vi "instert_before.vi"(8 "error in (no error)":errorcluster, 9 "current node":refnum<class "Iterator.lvclass">, 10 "data":variant, 11 "DoublyLinkedList in":refnum<class "DoublyLinkedList.lvclass">) -> (0 "error out":errorcluster, 3 "DoublyLinkedList out":refnum<class "DoublyLinkedList.lvclass">)   [LabVIEW 2021, in "DoublyLinkedList.lvclass"]
uses:
  DoublyLinkedList.lvclass
  Iterator/Iterator.lvclass
  DoublyLinkedList.lvclass/DoublyLinkedList.ctl
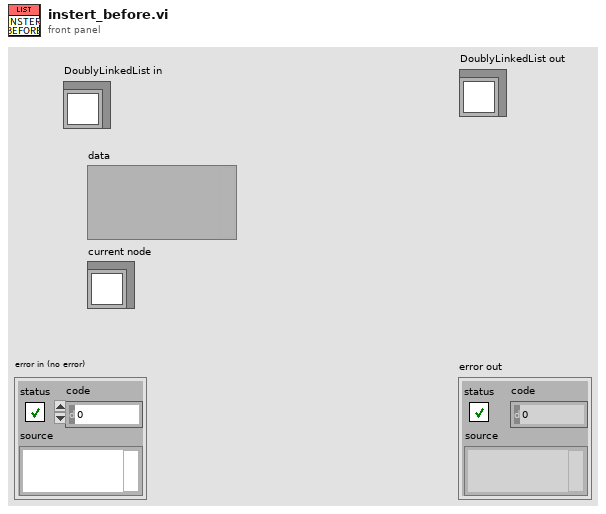
[diagram p1: front panel]
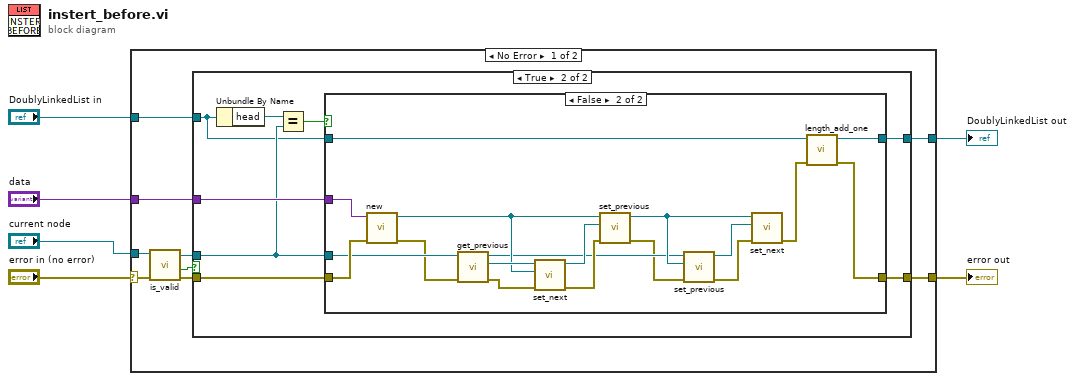
[diagram p0: block diagram]
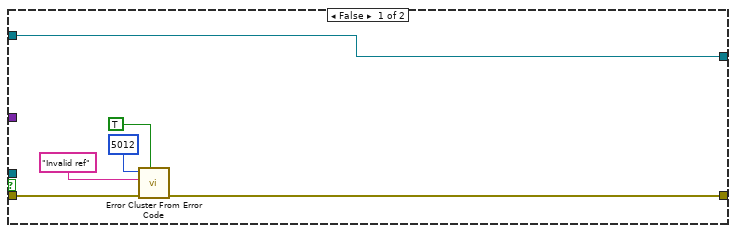
[diagram p2: hidden frame]
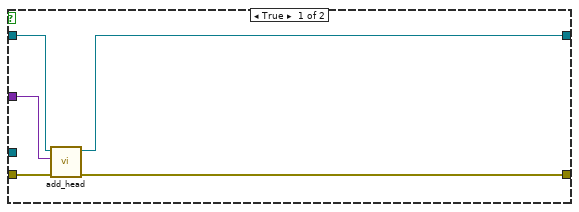
[diagram p3: hidden frame]
diagram:
  n1 = case shown="No Error" "error in (no error)" {
    selector: "error in (no error)" -> [w8 w54]
    tunnel: [w11 w54] -> w5
    tunnel: [w12 w53] -> w4
    tunnel: "data" -> [w13 _]
    tunnel: "current node" -> [w10 _]
    tunnel: "DoublyLinkedList in" -> [w14 w53]
    frame No Error {
      n2 = call-dynamic "is_valid.vi"("error in (no error)"=w8, "Iterator in"=w10) -> ("error out"=w7:errorcluster, "valid?"=w15:bool, "Iterator out"=w9:refnum<class "Iterator.lvclass">)  [unwired: 7 in]
      n3 = case shown="True" w15 {
        tunnel: w14 -> [w21 w23]
        tunnel: w13 -> [_ w29]
        tunnel: w7 -> [w18 w28]
        tunnel: w9 -> [_ w26]
        tunnel: [w21 w22] -> w12
        tunnel: [w17 w27] -> w11
        frame False {
          n4 = call <vilib>:"Error Cluster From Error Code.vi"("show call chain? (False)"=TRUE, "error in (no error)"=w18, "error message (\"\")"="Invalid ref" ("error message (\"\")"), "error code (0)"=5012) -> ("error out"=w17:errorcluster)  [unwired: 5 in]
        }
        frame True {
          n5 = Unbundle By Name(w23) -> ("head"=w25:refnum<class "Iterator.lvclass">)
          n6 = Equal?(x=w25, y=w26) -> (x = y?=w24:bool)
          n7 = case shown="False" w24 {
            tunnel: w28 -> [w33 w52]
            tunnel: w29 -> [w30 w51]
            tunnel: [w31 w35] -> w27
            tunnel: w26 -> [_ w50]
            tunnel: w23 -> [w34 w38]
            tunnel: [w32 w37] -> w22
            frame True {
              n8 = call-dynamic "add_head.vi"("error in (no error)"=w33, "data"=w30, "DoublyLinkedList in"=w34) -> ("error out"=w31:errorcluster, "DoublyLinkedList out"=w32:refnum<class "DoublyLinkedList.lvclass">)  [unwired: 7 in]
            }
            frame False {
              n9 = call "new.vi"("error in (no error)"=w52, "data"=w51) -> ("error out"=w49:errorcluster, "Iterator out"=w46:refnum<class "Iterator.lvclass">)  [unwired: 8 in]
              n10 = call-dynamic "get_previous.vi"("error in (no error)"=w49, "Iterator in"=w50) -> ("error out"=w45:errorcluster, "previous"=w48:refnum<class "Iterator.lvclass">, "Iterator out"=w40:refnum<class "Iterator.lvclass">)  [unwired: 6 in, 1 out]
              n11 = call-dynamic "set_next.vi"("error in (no error)"=w45, "next"=w46, "Iterator in"=w48) -> ("error out"=w41:errorcluster, "Iterator out"=w47:refnum<class "Iterator.lvclass">)  [unwired: 7 in]
              n12 = call-dynamic "set_previous.vi"("error in (no error)"=w41, "previous"=w47, "Iterator in"=w46) -> ("error out"=w39:errorcluster, "Iterator out"=w43:refnum<class "Iterator.lvclass">)  [unwired: 7 in]
              n13 = call-dynamic "set_previous.vi"("error in (no error)"=w39, "previous"=w43, "Iterator in"=w40) -> ("error out"=w42:errorcluster, "Iterator out"=w44:refnum<class "Iterator.lvclass">)  [unwired: 7 in]
              n14 = call-dynamic "set_next.vi"("error in (no error)"=w42, "next"=w44, "Iterator in"=w43) -> ("error out"=w36:errorcluster)  [unwired: 7 in, 1 out]
              n15 = call "length_add_one.vi"("error in (no error)"=w36, "DoublyLinkedList in"=w38) -> ("error out"=w35:errorcluster, "DoublyLinkedList out"=w37:refnum<class "DoublyLinkedList.lvclass">)  [unwired: 8 in]
            }
          }
        }
      }
    }
    frame Error {
    }
  }
  "error out" <- w5
  "DoublyLinkedList out" <- w4
